vi "Swap.vi"(8 "error in (no error)":errorcluster, 9 "size":u64 format="%d bytes", 10 "Pointer y":refnum<class "Pointer.lvclass">, 11 "Pointer x":refnum<class "Pointer.lvclass">) -> (0 "error out":errorcluster, 2 "Pointer y":refnum<class "Pointer.lvclass">, 3 "Pointer x":refnum<class "Pointer.lvclass">)   [LabVIEW 2027, in "Memory Manager.lvlib" / "Pointer.lvclass"]
doc: "Swaps <b>size</b> bytes between the sections of memory referred to by the two provided <b>Pointers</b>. The source and destination memory blocks should not overlap."
uses:
  Pointer.lvclass
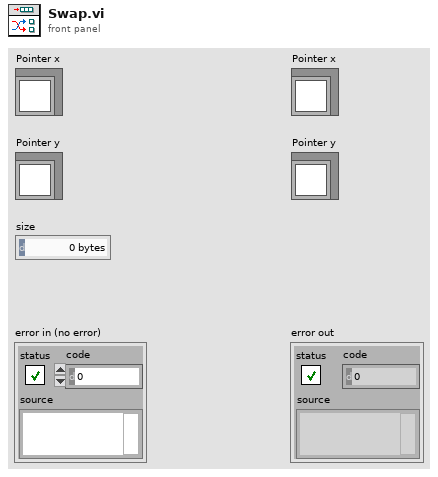
[diagram p1: front panel]
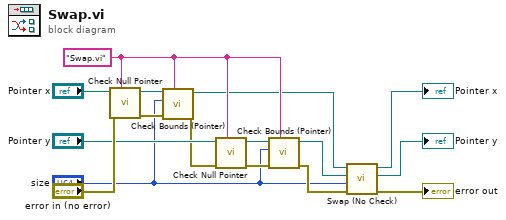
[diagram p0: block diagram]
diagram:
  w10 = "Swap.vi" ("source vi name")
  n1 = call "Check Null Pointer.vi"("source vi name"=w10, "error in (no error)"="error in (no error)", "Pointer in"="Pointer x") -> ("error out"=w9:errorcluster, "Pointer out"=w8:refnum<class "Pointer.lvclass">)  [unwired: 7 in]
  n2 = call "Check Bounds (Pointer).vi"("source vi name"=w10, "error in (no error)"=w9, "size"="size", "Pointer in"=w8) -> ("error out"=w5:errorcluster, "Pointer out"=w2:refnum<class "Pointer.lvclass">)  [unwired: 4 in, 2 out]
  n3 = call "Check Null Pointer.vi"("source vi name"=w10, "error in (no error)"=w5, "Pointer in"="Pointer y") -> ("error out"=w6:errorcluster, "Pointer out"=w7:refnum<class "Pointer.lvclass">)  [unwired: 7 in]
  n4 = call "Check Bounds (Pointer).vi"("source vi name"=w10, "error in (no error)"=w6, "size"="size", "Pointer in"=w7) -> ("error out"=w4:errorcluster, "Pointer out"=w3:refnum<class "Pointer.lvclass">)  [unwired: 4 in, 2 out]
  n5 = call "Swap (No Check).vi"("error in (no error)"=w4, "size"="size", "Pointer y"=w3, "Pointer x"=w2) -> ("error out"=→"error out":errorcluster, "Pointer y"=→"Pointer y":refnum<class "Pointer.lvclass">, "Pointer x"=→"Pointer x":refnum<class "Pointer.lvclass">)  [unwired: 5 in]
